vi "_session_set_additionalFlag_value.vi"(3 "New value in":bool, 4 "AdditionalFlag bit":T1, 5 "Additional Flags in":i32 format="%011b") -> (0 "Old value out":bool, 2 "Additional Flags out":i32 format="%011b")   [LabVIEW 2020, in "Rohde&Schwarz RTx Oscilloscopes.lvlib" / "rsidr_core.lvlib"]
doc: "OPC Timeout and VISA Timeout is not set if the 'int32 value in' is 0 or negative"
uses:
  rsidr_core.lvlib
  type_AdditionalFlag_Bits.ctl
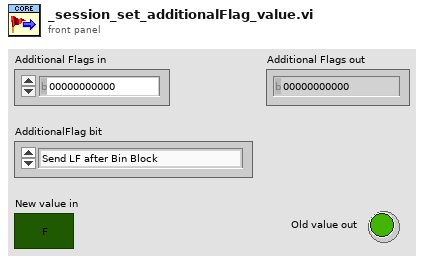
[diagram p1: front panel]
types:
  T1 = typedef "Rohde&Schwarz RTx Oscilloscopes.lvlib/rsidr_core.lvlib/type_AdditionalFlag_Bits.ctl" = enum16{"Send LF after Bin Block", "Junk read with io_clear_buffers.vi", "io_clear_buffers: viClear()", "io_clear_buffers: viFlush()", "<NotUsed1>", "Allow Dbl & Int Bin/Ascii read", "*OPC? in check_instrument_error.vi", "<NotUsed2>", "Smart Enum Matching", "Less Strict RepCaps check", "AssureResponseEndWithLF"}
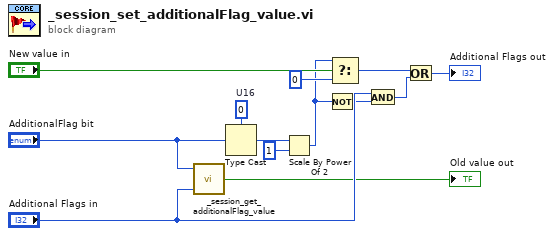
[diagram p0: block diagram]
diagram:
  w8 = u16 0  # U16
  n1 = call "_session_get_additionalFlag_value.vi"("AdditionalFlags value in"="Additional Flags in", "AdditionalFlag bit"="AdditionalFlag bit") -> ("AdditionalFlag bit value out"=→"Old value out":bool)  [unwired: 3 in]
  n2 = Type Cast(type=w8, x="AdditionalFlag bit") -> (*(type *) &x=w7:u16)
  n3 = Scale By Power Of 2(n=w7, x=1) -> (x*2^n=w5:i32)
  n4 = Not(x=w5) -> (.not. x?=w4:i32)
  n5 = Select(t=w5, s="New value in", f=0) -> (s? t:f=w3:i32)
  n6 = And(x="Additional Flags in", y=w4) -> (x .and. y?=w2:i32)
  n7 = Or(x=w3, y=w2) -> (x .or. y?=→"Additional Flags out":i32)
